vi "WIMDA data insert.vi"(8 "error in (no error)":errorcluster, 11 "WIMDA-data":T1) -> (0 "error out":errorcluster)   [LabVIEW 2016, in "AIRMAR WeatherCaster.lvlib"]
uses:
  AIRMAR WeatherCaster.lvlib
  NMEA_WIMDA-data.ctl
panel:
  in  "data in":T2
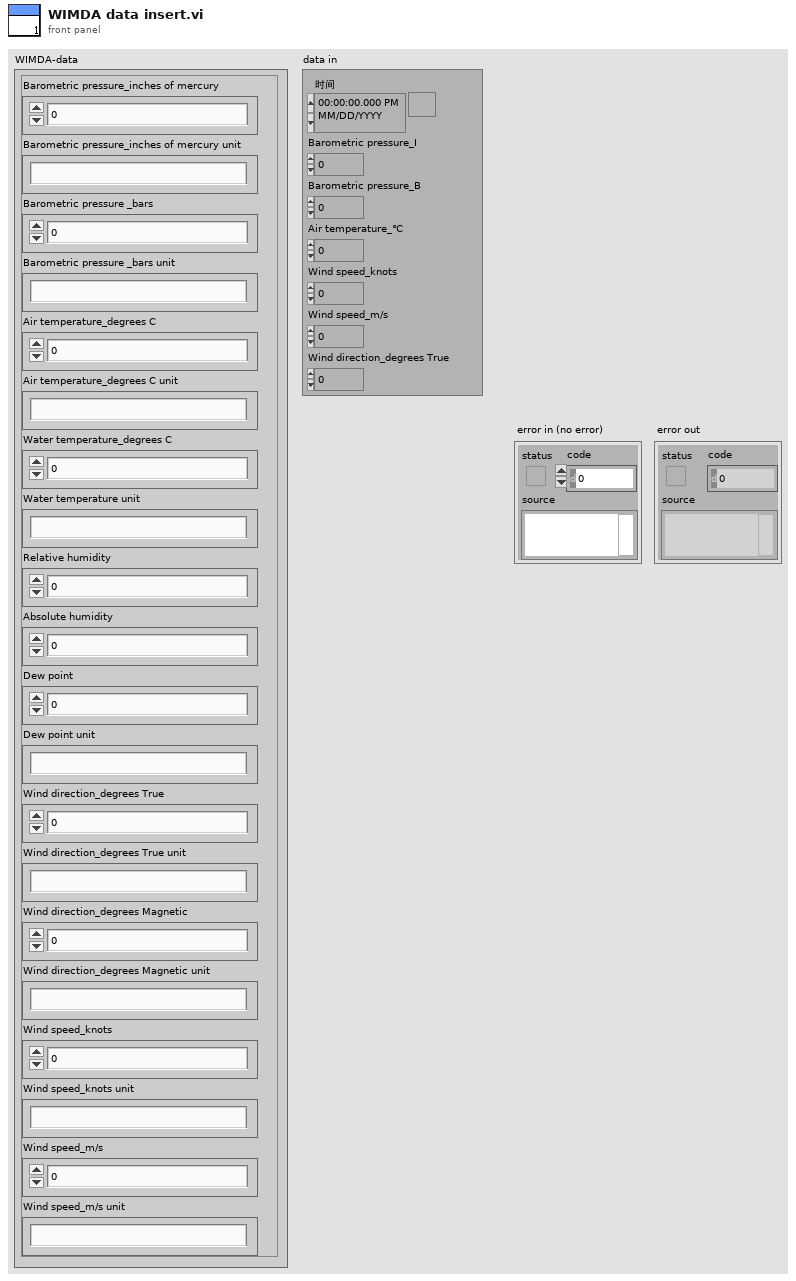
[diagram p1: front panel]
types:
  T1 = typedef "AIRMAR WeatherCaster.lvlib/NMEA_WIMDA-data.ctl" = cluster{"Barometric pressure_inches of mercury":dbl, "Barometric pressure_inches of mercury unit":string, "Barometric pressure _bars":dbl, "Barometric pressure _bars unit":string, "Air temperature_degrees C":dbl, "Air temperature_degrees C unit":string, "Water temperature_degrees C":dbl, "Water temperature unit":string, "Relative humidity":dbl, "Absolute humidity":dbl, "Dew point":dbl, "Dew point unit":string, "Wind direction_degrees True":dbl, "Wind direction_degrees True unit":string, "Wind direction_degrees Magnetic":dbl, "Wind direction_degrees Magnetic unit":string, "Wind speed_knots":dbl, "Wind speed_knots unit":string, "Wind speed_m/s":dbl, "Wind speed_m/s unit":string}
  T2 = cluster{"时间":timestamp, "Barometric pressure_I":dbl, "Barometric pressure_B":dbl, "Air temperature_℃":dbl, "Wind speed_knots":dbl, "Wind speed_m/s":dbl, "Wind direction_degrees True":dbl}
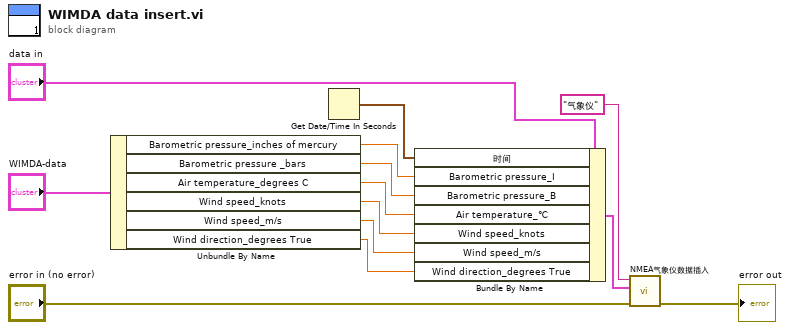
[diagram p0: block diagram]
diagram:
  n1 = Unbundle By Name("WIMDA-data") -> ("Barometric pressure_inches of mercury"=w10:dbl, "Barometric pressure _bars"=w9:dbl, "Air temperature_degrees C"=w8:dbl, "Wind speed_knots"=w7:dbl, "Wind speed_m/s"=w6:dbl, "Wind direction_degrees True"=w5:dbl)
  n2 = Get Date/Time In Seconds() -> (seconds since 1Jan1904=w11:timestamp)
  n3 = Bundle By Name(cluster="data in", "时间"=w11, "Barometric pressure_I"=w10, "Barometric pressure_B"=w9, "Air temperature_℃"=w8, "Wind speed_knots"=w7, "Wind speed_m/s"=w6, "Wind direction_degrees True"=w5) -> (w3:T2)
  n4 = call "NMEA气象仪数据插入.vi"("Tabe Name"="气象仪" ("table"), "data"=w3, "错误输入（无错误）"="error in (no error)") -> ("错误输出"=→"error out":errorcluster)  [unwired: 7 in]
